vi "Actor Core.vi"(8 "error in":errorcluster, 11 "Process State in":refnum<class "Process State.lvclass">) -> (0 "error out":errorcluster, 3 "Actor out":refnum<class "Actor.lvclass">)   [LabVIEW 2013, in "Process States.lvlib" / "Process State.lvclass"]
doc: "(<B>Filename</B>: Actor Framework.lvlib:Actor.lvclass:Actor Core.vi)\n\n\nThis override launches an instance of Process Actor.lvclass.\n\nReceives messages to the actor, reacts to them, and initiates any error handling that may shut the actor down.\n\nDescendant classes may override this VI to append parallel tasks for the actor to complete while it handles messages. Overrides use the Call Parent Method node."
uses:
  Process State.lvclass
  <vilib>/ActorFramework/Actor/Actor.lvclass
  Process Actor/Process/Process.lvclass
  <vilib>/ActorFramework/Actor/Actor.lvclass/Actor.ctl
  <vilib>/ActorFramework/Message Enqueuer/Message Enqueuer.lvclass/Message Enqueuer.ctl
  Process State.lvclass/Process State.ctl
  State Actor/State Actor.lvclass
  <vilib>/ActorFramework/Message Enqueuer/Init from Existing Queue.vi
  <vilib>/ActorFramework/Message Enqueuer/Message Enqueuer.lvclass
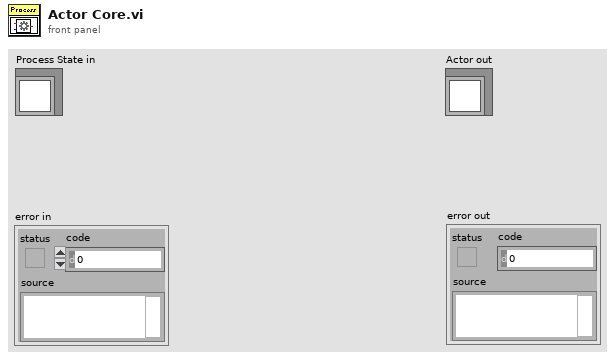
[diagram p1: front panel]
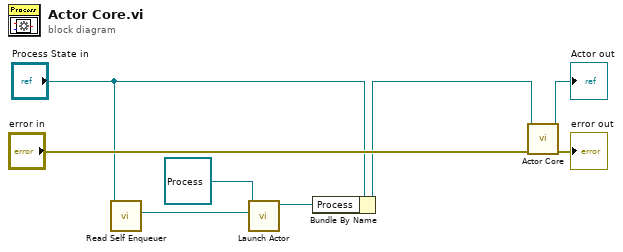
[diagram p0: block diagram]
diagram:
  n1 = call <vilib>:"Read Self Enqueuer.vi"("Actor"="Process State in") -> ("Self Enqueuer"=w6:refnum<class "Message Enqueuer.lvclass">)  [unwired: 10 in]
  n2 = call <vilib>:"Launch Actor.vi"("Actor-to-Caller Enqueuer"=w6, "Actor"=refnum<class "Process.lvclass"> refnum ("Process Actor.lvlib:Process.lvclass")) -> ("Caller-To-Actor Enqueuer"=w4:refnum<class "Message Enqueuer.lvclass">)  [unwired: 8 in, 1 out]
  n3 = Bundle By Name(cluster="Process State in", "Process"=w4) -> (w2:refnum<class "Process State.lvclass">)
  n4 = call-parent "Actor Core.vi"("error in"="error in", "State in"=w2) -> ("error out"=→"error out":errorcluster, "Actor out"=→"Actor out":refnum<class "Actor.lvclass">)  [unwired: 8 in]
